vi "Read Write Text File.vi"(0 "File Path":path=path "C:/Projects/labview_tips_2024/src/Assessment01/TextFile.txt", 5 "File Operation":T1, 7 "Text Input":string, 11 "Error In":errorcluster) -> (4 "Text Output":string, 15 "Error Out":errorcluster)   [LabVIEW 2023, in "File and Path Operations.lvlib"]
doc: "This VI can read from and write to a specified text file based on the selected operation mode."
uses:
  File and Path Operations.lvlib
  Controls/FileOperation.ctl
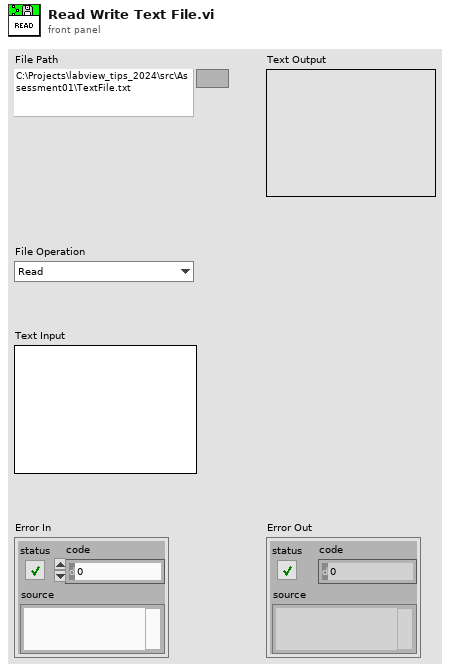
[diagram p1: front panel]
types:
  T1 = typedef "File and Path Operations.lvlib/FileOperation.ctl" = enum16{"Read", "Write"}
  T2 = enum16{"open", "replace", "create", "open or create", "replace or create", "replace or create with confirmation"}
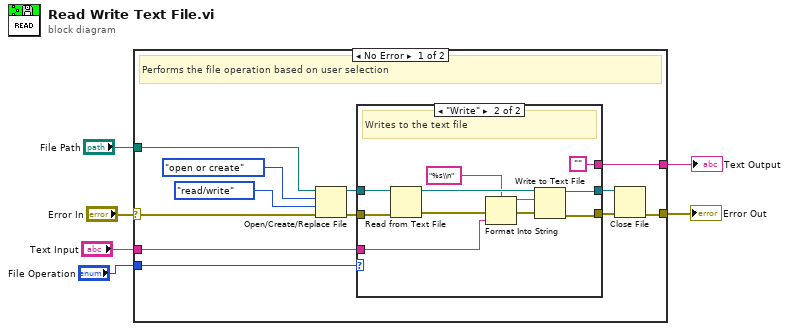
[diagram p0: block diagram]
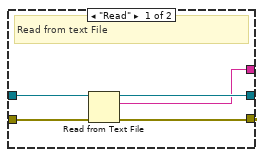
[diagram p2: hidden frame]
diagram:
  n1 = case shown="No Error" "Error In" {
    selector: "Error In" -> [w14 w35]
    tunnel: [w18 w35] -> w1
    tunnel: [w15 _] -> w5
    tunnel: "File Path" -> [w10 _]
    tunnel: "File Operation" -> [w9 _]
    tunnel: "Text Input" -> [w8 _]
    frame No Error {
      # "Performs the file operation based on user selection"
      n2 = Open/Create/Replace File(file path (use dialog)=w10, error in=w14, operation (0:open)=T2."open or create", access (0:read/write)=enum16{"read/write", "read-only", "write-only"}."read/write") -> (refnum out=w12:refnum<file>, error out=w11:errorcluster)  [unwired: 2 in, 1 out]
      n3 = case shown="\"Write\"" w9 {
        tunnel: w12 -> [w23 w30]
        tunnel: w11 -> [w22 w33]
        tunnel: [w19 ""] -> w15
        tunnel: [w21 w32] -> w17
        tunnel: [w20 w34] -> w16
        tunnel: w8 -> [_ w25]
        frame "Read" {
          # "Read from text File"
          n4 = Read from Text File(file (use dialog)=w23, error in=w22) -> (refnum out=w20:refnum<file>, text=w19:string, error out=w21:errorcluster)  [unwired: 2 in, 1 out]
        }
        frame "Write" {
          # "Writes to the text file"
          n5 = Read from Text File(file (use dialog)=w30, error in=w33) -> (refnum out=w31:refnum<file>, error out=w28:errorcluster)  [unwired: 2 in, 2 out]
          n6 = Format Into String(format string="%s\\n", error in=w28, w25) -> (resulting string=w26:string, error out=w27:errorcluster)  [unwired: 1 in]
          n7 = Write to Text File(file (use dialog)=w31, text=w26, error in=w27) -> (refnum out=w34:refnum<file>, error out=w32:errorcluster)  [unwired: 1 in, 1 out]
        }
      }
      n8 = Close File(refnum=w16, error in=w17) -> (error out=w18:errorcluster)  [unwired: 1 out]
    }
    frame Error {
      # "Returns the default values"
    }
  }
  "Text Output" <- w5
  "Error Out" <- w1
